vi "CreateGUI.vi"(8 "ErrorIn":errorcluster, 11 "GUIs":T2(array[cluster])) -> (0 "ErrorOut":errorcluster, 3 "TAFProjDocumentType:FrontPanelGUIOut":refnum<class "FrontPanelGUI.lvclass">)   [LabVIEW 2021, in "TAF Proj Document Type.lvlib" / "FrontPanelGUI.lvclass"]
uses:
  <vilib>/Wovalab/AntiDoc/Document Type/Add-ons/LabVIEW TAF Project/FrontPanelGUI/FrontPanelGUI.lvclass
  C:/Program Files (x86)/National Instruments/LabVIEW 2021/vi.lib/Wovalab/AntiDoc/Bloc/Bloc.lvclass
  <vilib>/picture/picture.llb/imagedata.ctl
  <vilib>/Wovalab/AntiDoc/Bloc/Bloc.lvclass/Bloc.ctl
  <vilib>/Wovalab/AntiDoc/Document Type/Add-ons/LabVIEW TAF Project/FrontPanelGUI/FrontPanelGUI.lvclass/FrontPanelGUI.ctl
  <vilib>/Wovalab/AntiDoc/Bloc/Write Name.vi
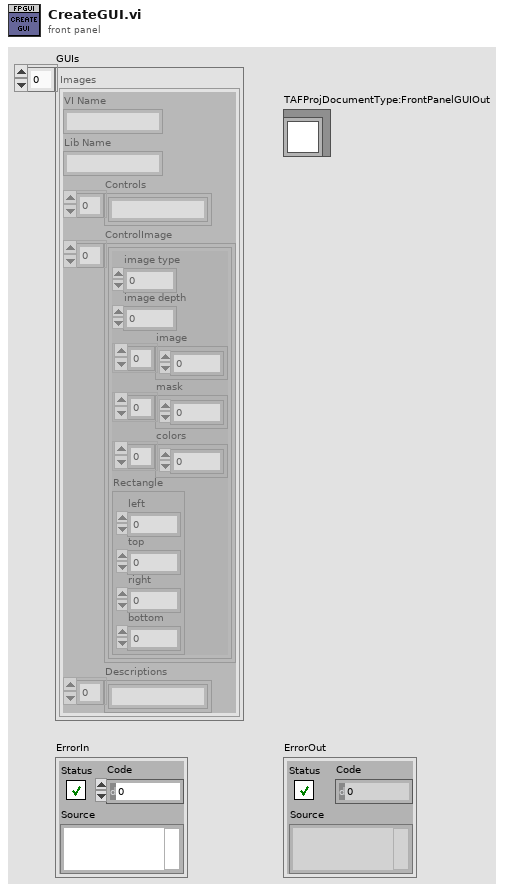
[diagram p1: front panel]
types:
  T1 = typedef "imagedata.ctl" = cluster{"image type":i32, "image depth":i32, "image":u8[], "mask":u8[], "colors":u32[], "Rectangle":cluster{"left":i16, "top":i16, "right":i16, "bottom":i16}}
  T2 = cluster{"VI Name":string, "Lib Name":string, "Controls":string[], "ControlImage":T1[], "Descriptions":string[]}[]
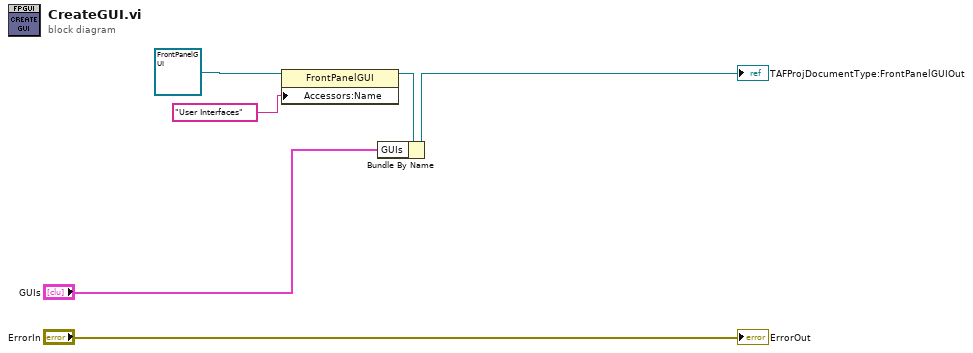
[diagram p0: block diagram]
diagram:
  n1 = property class="FrontPanelGUI"(reference=refnum<class "FrontPanelGUI.lvclass"> refnum ("TAF Proj Document Type.lvlib:FrontPanelGUI"), "Accessors:Name"="User Interfaces" ("Name")) -> (reference out=w4:refnum<class "FrontPanelGUI.lvclass">)  [unwired: 1 in, 1 out]
  n2 = Bundle By Name(cluster=w4, "GUIs"="GUIs") -> (→"TAFProjDocumentType:FrontPanelGUIOut":refnum<class "FrontPanelGUI.lvclass">)
  "ErrorOut" <- "ErrorIn"
